vi "Komponent Konzentration mit Name finden.vi"(10 "Konzentration IST in":dbl, 11 "Komponente":string) -> (1 "found":bool, 2 "Konzentration OUT":dbl, 3 "Gasauswahl":string)   [LabVIEW 2020, in "System Einstellungen V2.lvlib"]
uses:
  System Einstellungen V2.lvlib
  Aktion FGV Gasbottledefinition.ctl
  <vilib>/regexp/Match Regular Expression.xnode
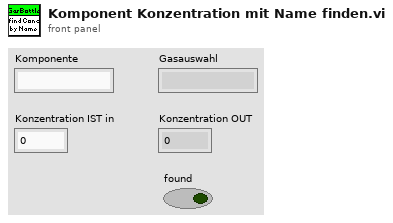
[diagram p1: front panel]
types:
  T1 = typedef "System Einstellungen V2.lvlib/Aktion FGV Gasbottledefinition.ctl" = enum16{"lesen", "schreiben", "löschen", "laden", "speichern", "exportieren", "importieren"}
  T2 = typedef "System Einstellungen V2.lvlib/Gasflasche gesamt.ctl" = cluster{"Gasflasche":T3, "Trägergas":T4, "Komponenten":T5[]}
  T3 = typedef "System Einstellungen V2.lvlib/Gasflasche.ctl" = cluster{"Gasname für die Auswahl":string, "Chargennummer":string, "Ablaufdatum":timestamp}
  T4 = typedef "System Einstellungen V2.lvlib/Traegergas.ctl" = string
  T5 = typedef "System Einstellungen V2.lvlib/Gasflaschenkomponente.ctl" = cluster{"Gasauswahl":string, "Konzentration IST":dbl, "Einheit":string, "Genauigkeit":dbl}
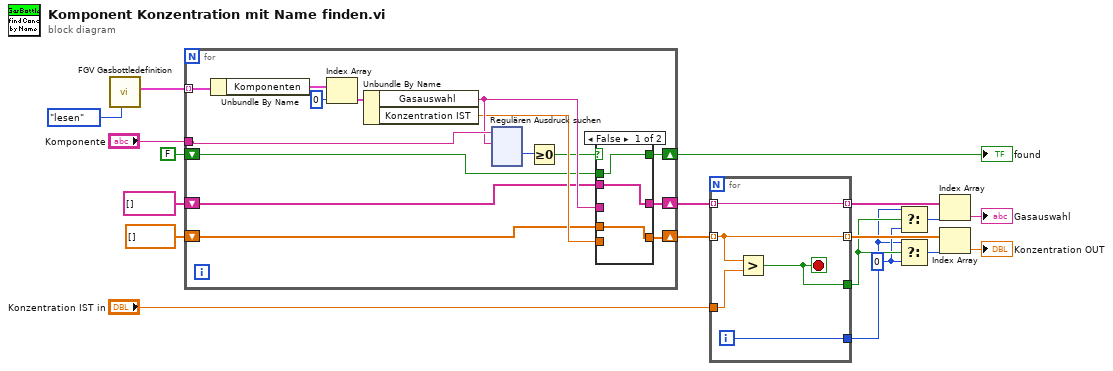
[diagram p0: block diagram]
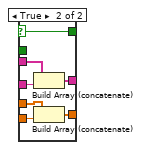
[diagram p2: hidden frame]
diagram:
  w2 = 0 ("f")
  n1 = call "FGV Gasbottledefinition.vi"("Aktion"=Aktion_FGV_Gasbottledefinition."lesen") -> ("Gasflaschen Liste gesamt"=w18:T2[])  [unwired: 8 in, 2 out]
  n2 = for {
    tunnel: w18 -> [w34] mode=indexing
    tunnel: "Komponente" -> [w29]
    shift-right: [w26] -> w14
    shift-left: string[] [] -> [w24]
    shift-right: [w25] -> w13
    shift-left: dbl[] [] -> [w23]
    shift-right: [w21] -> w11
    shift-left: FALSE -> [w20]
    n3 = Unbundle By Name(w34) -> ("Komponenten"=w33:T5[])
    n4 = Index Array(array=w33, index=0 ("Index")) -> (element=w32:T5)
    n5 = Unbundle By Name(w32) -> ("Gasauswahl"=w28:string, "Konzentration IST"=w27:dbl)
    n6 = xnode "Regulären Ausdruck suchen"("Eingangs-String"=w29, "Regulärer Ausdruck"=w28) -> ("Offset nach Übereinstimmung"=w31:i32)  [unwired: 4 in, 4 out]
    n7 = Greater Or Equal To 0?(x=w31) -> (x >= 0?=w22:bool)
    n8 = case shown="False" w22 {
      selector: w22 -> [_ w38]
      tunnel: w28 -> [_ w44]
      tunnel: w27 -> [_ w43]
      tunnel: [w37 w42] -> w26
      tunnel: [w36 w41] -> w25
      tunnel: w24 -> [w37 w40]
      tunnel: w23 -> [w36 w39]
      tunnel: [w35 w38] -> w21
      tunnel: w20 -> [w35 _]
      frame False {
      }
      frame True {
        n9 = Build Array (concatenate)(w40, w44) -> (w42:string[])
        n10 = Build Array (concatenate)(w39, w43) -> (w41:dbl[])
      }
    }
  }
  "found" <- w11
  n11 = for {
    tunnel: w14 -> [w161] mode=indexing
    tunnel: w13 -> [w162] mode=indexing
    tunnel: "Konzentration IST in" -> [w163]
    tunnel: [w162] -> w7 mode=indexing
    tunnel: [w161] -> w8 mode=indexing
    tunnel: [w160] -> w3
    tunnel: [w159] -> w1
    i -> [w159]
    stop <- w160 stop-if-true
    n12 = Greater?(x=w162, y=w163) -> (0:w160:bool)
  }
  n13 = Select(t=w1, s=w3, f=w2) -> (s? t:f=w4:i32)
  n14 = Select(t=w1, s=w3, f=w2) -> (s? t:f=w5:i32)
  n15 = Index Array(array=w8, index=w4) -> (element=→"Gasauswahl":string)
  n16 = Index Array(array=w7, index=w5) -> (element=→"Konzentration OUT":dbl)
